vi "读取数据文件.vi"(8 "错误输入（无错误）":errorcluster, 11 "数据文件路径":path) -> (0 "错误输出":errorcluster, 3 "数据":T1[](array[typedef]))   [LabVIEW 2020]
uses:
  <vilib>/drjdpowell/SQLite Library/SQL Statement/SQL Statement.lvclass/SQL Statement.ctl
  <vilib>/drjdpowell/SQLite Library/SQL Connection/Open (path).vi
  <vilib>/drjdpowell/SQLite Library/SQL Statement/Column I64.vi
  <vilib>/drjdpowell/SQLite Library/SQL Connection/Open (string).vi
  <vilib>/AdvancedString/Path To Command Line String.vi
  <vilib>/drjdpowell/SQLite Library/SQL Statement/Error Message.vi
  <vilib>/drjdpowell/SQLite Library/SQL Statement/Column Timestamp.vi
  <vilib>/drjdpowell/SQLite Library/SQL Statement/Column String.vi
  <vilib>/drjdpowell/SQLite Library/SQL Connection/Connection.lvclass
  <vilib>/drjdpowell/SQLite Library/SQL Statement/SQL Statement.lvclass
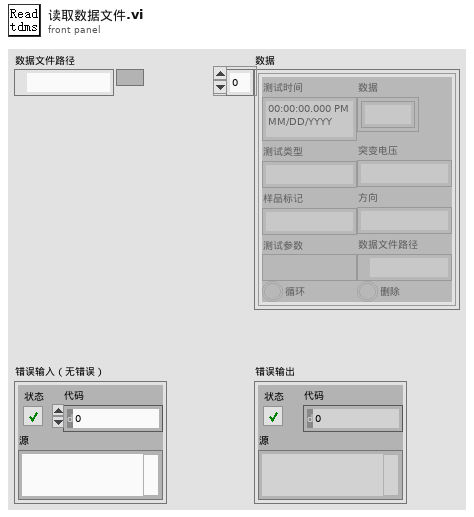
[diagram p1: front panel]
types:
  T1 = typedef "测试数据类型.ctl" = cluster{"测试时间":timestamp, "测试类型":string, "样品标记":string, "测试参数":variant, "循环":bool, "数据":dbl[][], "删除":bool, "突变电压":i32, "方向":string, "数据文件路径":path}
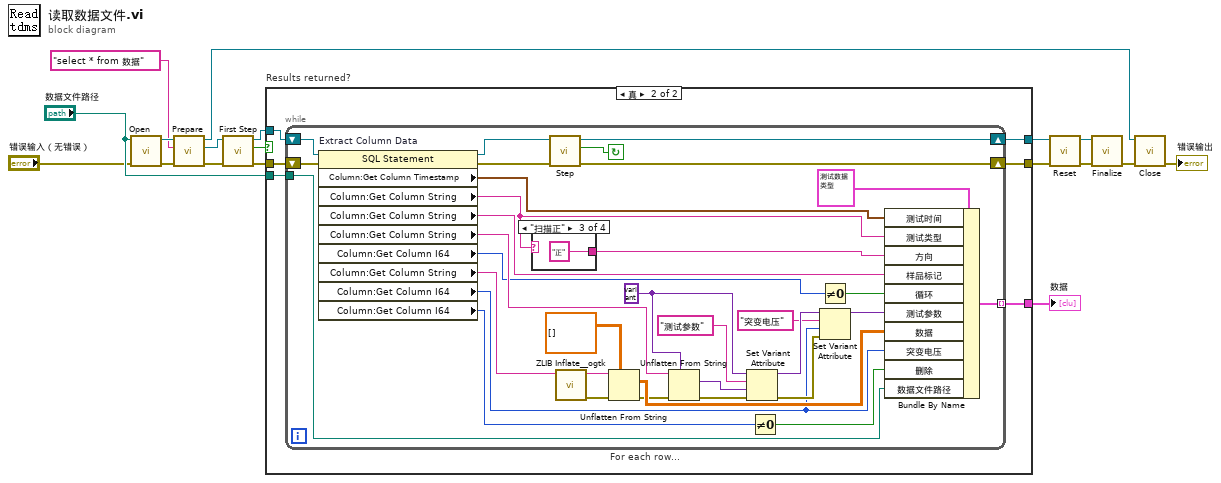
[diagram p0: block diagram]
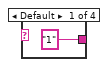
[diagram p3: hidden frame]
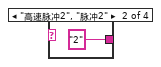
[diagram p4: hidden frame]
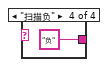
[diagram p5: hidden frame]
diagram:
  n1 = call-poly <vilib>:"Open.vi"("error in (no error)"="错误输入（无错误）", "db file"="数据文件路径") -> ("error out"=w12:errorcluster, "SQLite Connection"=w10:refnum<class "Connection.lvclass">)  [unwired: 8 in]
  n2 = call <vilib>:"Prepare.vi"("error in (no error)"=w12, "SQL"="select * from 数据", "SQLite Connection in"=w10) -> ("error out"=w11:errorcluster, "SQL Statement"=w13:refnum<class "SQL Statement.lvclass">, "SQLite Connection"=w9:refnum<class "Connection.lvclass">)  [unwired: 4 in, 2 out]
  n3 = call <vilib>:"First Step.vi"("error in (no error)"=w11, "SQL Statement in"=w13) -> ("error out"=w15:errorcluster, "Row returned"=w14:bool, "SQL Statement"=w16:refnum<class "SQL Statement.lvclass">)  [unwired: 7 in]
  n4 = case "Results returned?" shown="真" w14 {
    tunnel: [w20 w26] -> w17
    tunnel: [w19 w25] -> w18
    tunnel: w16 -> [w20 w24]
    tunnel: w15 -> [w19 w23]
    tunnel: "数据文件路径" -> [_ w22]
    tunnel: [_ w21] -> w5
    frame False {
    }
    frame True {
      n5 = while "For each row..." {
        shift-right: [w59] -> w26
        shift-left: w24 -> [w56]
        shift-right: [w57] -> w25
        shift-left: w23 -> [w55]
        tunnel: w22 -> [w40]
        tunnel: [w39] -> w21 mode=indexing
        stop <- w54 continue-if-true
        w47 = variant ("变体")
        n6 = property on="Extract Column Data" class="SQL Statement"(reference=w56, error in=w55) -> (reference out=w60:refnum<class "SQL Statement.lvclass">, error out=w58:errorcluster, "Column:Get Column Timestamp"=w52:timestamp, "Column:Get Column String"=w41:string, "Column:Get Column String"=w51:string, "Column:Get Column String"=w50:string, "Column:Get Column I64"=w49:i64, "Column:Get Column String"=w45:string, "Column:Get Column I64"=w28:i64, "Column:Get Column I64"=w29:i64)
        n7 = case shown="\"扫描正\"" w41 {
          tunnel: ["1" ("名称") "2" ("名称") "正" ("名称") "负" ("名称")] -> w38
          frame Default {
          }
          frame "高速脉冲2", "脉冲2" {
          }
          frame "扫描正" {
          }
          frame "扫描负" {
          }
        }
        n8 = call <vilib>:"Step.vi"("error in (no error)"=w58, "SQL Statement in"=w60) -> ("error out"=w57:errorcluster, "Row returned"=w54:bool, "SQL Statement"=w59:refnum<class "SQL Statement.lvclass">)  [unwired: 7 in]
        n9 = call <userlib>:"ZLIB Inflate__ogtk.vi"("input"=w45) -> ("error out"=w36:errorcluster, "inflated output"=w44:string)  [unwired: 4 in, 1 out]
        n10 = Unflatten From String(type=dbl[][] [], binary string=w44, error in (no error)=w36) -> (value=w42:dbl[][], error out=w35:errorcluster)  [unwired: 2 in, 1 out]
        n11 = Unflatten From String(type=w47, binary string=w50, error in (no error)=w35) -> (value=w48:variant, error out=w37:errorcluster)  [unwired: 2 in, 1 out]
        n12 = Set Variant Attribute(Variant=w47, name="测试参数" ("元素"), value=w48, error in=w37) -> (Variant out=w33:variant, error out=w30:errorcluster)  [unwired: 1 out]
        n13 = Not Equal To 0?(x=w29) -> (x != 0?=w27:bool)
        n14 = Not Equal To 0?(x=w49) -> (x != 0?=w34:bool)
        n15 = Set Variant Attribute(Variant=w33, name="突变电压" ("名称"), value=w28, error in=w30) -> (Variant out=w32:variant)  [unwired: 2 out]
        n16 = Bundle By Name(cluster=T1 {"测试时间"=timestamp(0 s since 1904-01-01), "测试类型"="", "样品标记"="", "测试参数"=variant(string ""), "循环"=FALSE, "数据"=[], "删除"=FALSE, "突变电压"=0, "方向"="", "数据文件路径"=path ""} ("测试数据"), "测试时间"=w52, "测试类型"=w41, "方向"=w38, "样品标记"=w51, "循环"=w34, "测试参数"=w32, "数据"=w42, "突变电压"=w28, "删除"=w27, "数据文件路径"=w40) -> (w39:T1)
      }
    }
  }
  "数据" <- w5
  n17 = call <vilib>:"Reset.vi"("error in (no error)"=w18, "SQL Statement in"=w17) -> ("error out"=w8:errorcluster, "SQL Statement"=w1:refnum<class "SQL Statement.lvclass">)  [unwired: 8 in]
  n18 = call <vilib>:"Finalize.vi"("error in (no error)"=w8, "SQL Statement in"=w1) -> ("error out"=w2:errorcluster)  [unwired: 9 in]
  n19 = call-dynamic "Close.vi"("error in (no error)"=w2, "SQLite Connection in"=w9) -> ("error out"=→"错误输出":errorcluster)  [unwired: 9 in]
